vi "MALT132_003_OneCommand_OnOffInOneSec.vi"() -> ()   [LabVIEW 2018]
panel:
  out "x-y":u32
  out "Off &  On Cycles":i32
  in  "stop":bool
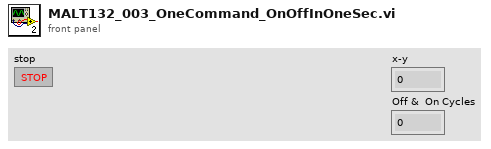
[diagram p1: front panel]
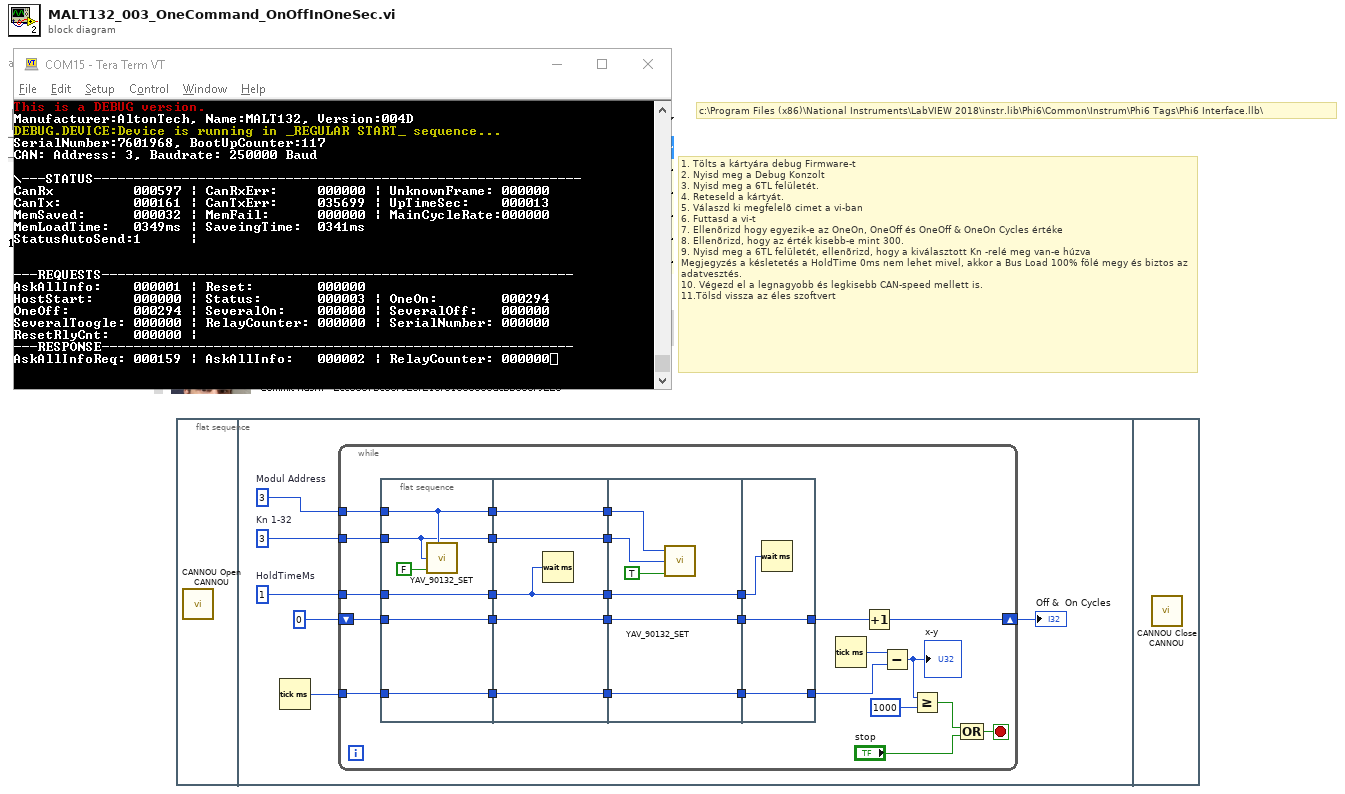
[diagram p0: block diagram]
diagram:
  # "1. Tölts a kártyára debug Firmware-t\n2. Nyisd meg a Debug Konzolt\n3. Nyisd meg a 6TL felületét.\n4. Reteseld a kártyát.\n5. Válaszd ki megfelelõ cimet a vi-ban\n6. Futtasd a vi-t\n7. Ellenõrizd hogy egyezik-e az OneOn, OneOff és OneOff & OneOn Cycles értéke\n8. Ellenõrizd, hogy az érték kisebb-e mint 300.\n9. Nyisd meg a 6TL felületét, ellenõrizd, hogy a kiválasztott Kn -relé meg van-e húzva\nMegjegyzés a késletetés a HoldTime 0ms nem lehet mivel, akkor a Bus Load 100% fölé megy és biztos az adatvesztés.\n10. Végezd el a legnagyobb és legkisebb CAN-speed mellett is.\n11.Tölsd vissza az éles szoftvert"
  # "c:\\Program Files (x86)\\National Instruments\\LabVIEW 2018\\instr.lib\\Phi6\\Common\\Instrum\\Phi6 Tags\\Phi6 Interface.llb\\"
  n1 = flat-sequence {
    frame #0 {
      n2 = call <instrlib>:"CANNOU Open CANNOU.vi"() -> ()  [unwired: 6 in, 2 out]
    }
    frame #1 {
      w6 = u8 3  # Modul Address
      w5 = u8 3  # Kn 1-32
      w1 = 1  # HoldTimeMs
      n3 = Tick Count (ms)() -> (millisecond timer value=w2:u32)
      n4 = while {
        tunnel: w6 -> [w33]
        tunnel: w5 -> [w28]
        shift-right: [w21] -> w3
        shift-left: 0 -> [w25]
        tunnel: w2 -> [w20]
        tunnel: w1 -> [w9]
        stop <- w13 stop-if-true
        n5 = flat-sequence {
          tunnel: w33 -> [w39]
          tunnel: [w39] -> w32
          tunnel: [w35] -> w30
          tunnel: w28 -> [w37]
          tunnel: [w37] -> w26
          tunnel: w25 -> [w36]
          tunnel: [w36] -> w23
          tunnel: w20 -> [w35]
          tunnel: [w34] -> w10
          tunnel: w9 -> [w34]
          tunnel: w32 -> [w44]
          tunnel: [w44] -> w31
          tunnel: w30 -> [w43]
          tunnel: [w43] -> w29
          tunnel: [w42] -> w27
          tunnel: w26 -> [w42]
          tunnel: [w41] -> w24
          tunnel: w23 -> [w41]
          tunnel: w10 -> [w40]
          tunnel: [w40] -> w8
          tunnel: w31 -> [w49]
          tunnel: w29 -> [w46]
          tunnel: w27 -> [w48]
          tunnel: w24 -> [w47]
          tunnel: [w47] -> w12
          tunnel: [w46] -> w11
          tunnel: w8 -> [w45]
          tunnel: [w45] -> w7
          tunnel: [w52] -> w18
          tunnel: [w53] -> w22
          tunnel: w12 -> [w53]
          tunnel: w11 -> [w52]
          tunnel: w7 -> [w51]
          frame #0 {
            n6 = call "YAV_90132_SET.vi"("Address"=w39, "Relay Num"=w37, "State"=FALSE) -> ()  [unwired: 2 in, 1 out]
          }
          frame #1 {
            n7 = Wait (ms)(milliseconds to wait=w40) -> ()  [unwired: 1 out]
          }
          frame #2 {
            n8 = call "YAV_90132_SET.vi"("Address"=w49, "Relay Num"=w48, "State"=TRUE) -> ()  [unwired: 2 in, 1 out]
          }
          frame #3 {
            n9 = Wait (ms)(milliseconds to wait=w51) -> ()  [unwired: 1 out]
          }
        }
        n10 = Tick Count (ms)() -> (millisecond timer value=w19:u32)
        n11 = Increment(x=w22) -> (x+1=w21:i32)
        n12 = Subtract(x=w19, y=w18) -> (x-y=w17:u32)
        "x-y" <- w17
        n13 = Greater Or Equal?(x=w17, y=u32 1000) -> (x >= y?=w15:bool)
        n14 = Compound Arithmetic op=OR(w15, "stop") -> (w13:bool)
      }
      "Off &  On Cycles" <- w3
    }
    frame #2 {
      n15 = call <instrlib>:"CANNOU Close CANNOU.vi"() -> ()  [unwired: 7 in, 1 out]
    }
  }
